vi "WriteVariable.vi"(8 "error in (no error)":errorcluster, 9 "ns":i32=2, 10 "variable_node":string, 11 "Server in":refnum<class "Server.lvclass">) -> (0 "error out":errorcluster, 3 "Server out":refnum<class "Server.lvclass">)   [LabVIEW 2017, in "opcua.lvlib" / "Server.lvclass"]
uses:
  Server.lvclass
  Server.lvclass/Server.ctl
  opcua32.dll
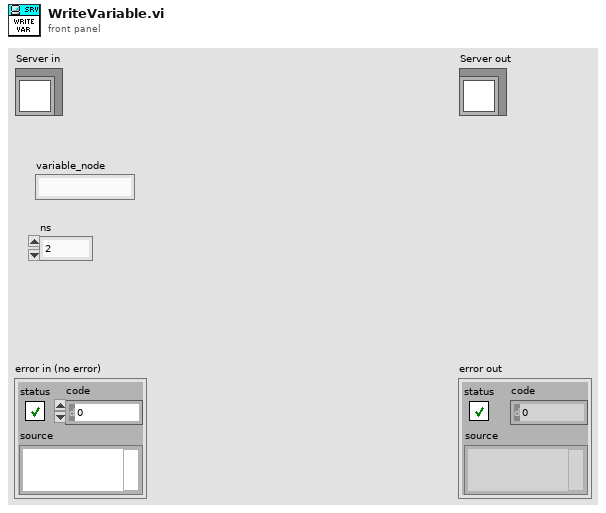
[diagram p1: front panel]
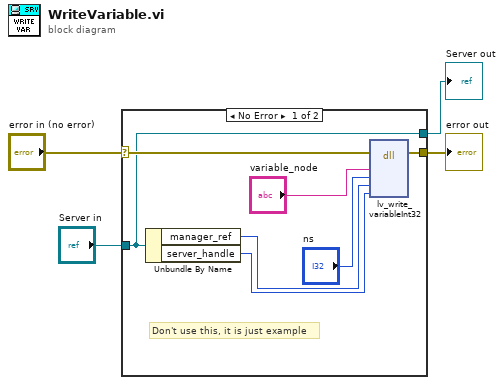
[diagram p0: block diagram]
diagram:
  n1 = case shown="No Error" "error in (no error)" {
    selector: "error in (no error)" -> [w10 w12]
    tunnel: [w9 w12] -> w3
    tunnel: [w5 w13] -> w1
    tunnel: "Server in" -> [w5 w13]
    frame No Error {
      # "Don't use this, it is just example"
      n2 = Unbundle By Name(w5) -> ("manager_ref"=w11:u64, "server_handle"=w6:u64)
      n3 = dll-call lib="C:/Users/Andrey/Desktop/opcua-labview/opcua-lvlib/opcua*.dll" fn="lv_write_variableInt32"(error in=w10, "variable_node"="variable_node", "ns"="ns", "manager"=w11, "handle"=w6) -> (error out=w9:errorcluster)  [unwired: 7 in, 1 out]
    }
    frame Error {
    }
  }
  "error out" <- w3
  "Server out" <- w1
